vi "LibreVNA Test 03.vi"() -> ()   [LabVIEW 2023]
uses:
  LibreVNA/LibreVNA.lvclass
panel:
  in  "Run":bool
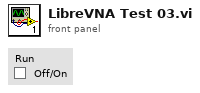
[diagram p1: front panel]
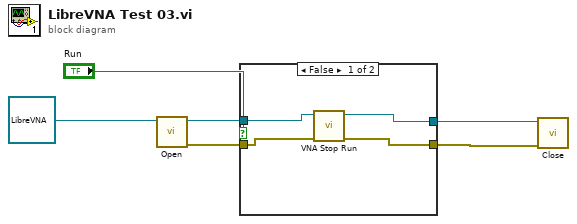
[diagram p0: block diagram]
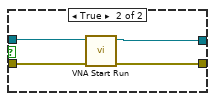
[diagram p2: hidden frame]
diagram:
  n1 = call-dynamic "Open.vi"("LibreVNA in"=refnum<class "LibreVNA.lvclass"> refnum ("LibreVNA.lvclass")) -> ("error out"=w4:errorcluster, "LibreVNA out"=w5:refnum<class "LibreVNA.lvclass">)  [unwired: 9 in]
  n2 = case shown="False" "Run" {
    tunnel: w5 -> [w10 w14]
    tunnel: w4 -> [w9 w13]
    tunnel: [w7 w12] -> w3
    tunnel: [w8 w11] -> w2
    frame False {
      n3 = call-dynamic "VNA Stop Run.vi"("error in (no error)"=w9, "LibreVNA in"=w10) -> ("error out"=w8:errorcluster, "LibreVNA out"=w7:refnum<class "LibreVNA.lvclass">)  [unwired: 7 in, 1 out]
    }
    frame True {
      n4 = call-dynamic "VNA Start Run.vi"("error in (no error)"=w13, "LibreVNA in"=w14) -> ("error out"=w11:errorcluster, "LibreVNA out"=w12:refnum<class "LibreVNA.lvclass">)  [unwired: 7 in, 1 out]
    }
  }
  n5 = call-dynamic "Close.vi"("error in (no error)"=w2, "LibreVNA in"=w3) -> ()  [unwired: 8 in, 2 out]
